vi "Interpolate (single).vi"(8 "error in (no error)":errorcluster, 10 "Configure":T1={"X Low"=0.05, "X High"=0.5, "X Step"=0.01, "Fake Point"=0.05} {"Fake Point" format="%#_6p"; "X Step" format="%#_6p"; "X High" format="%#_6p"; "X Low" format="%#_6p"}, 11 "XY-data":cluster{"X-array":dbl[], "Y-array":dbl[]} {"Y-array" format="%#_6p"}) -> (0 "error out":errorcluster, 3 "Interpolated XY-data out":cluster{"X-array":dbl[], "Y-array":dbl[]} {"Y-array" format="%.2p"; "X-array" format="%.2p"})   [LabVIEW 2019, in "xy_utilities.lvlib"]
doc: "Use this VI to interpolate data and add \"fake\" points outside of the given x array.\n\nThe <b>Configure</b> cluster is used to define:\n<b>X Low</b>: Starting x value for interpolation. May lie outside of the input x array range.\n<b>X High</b>: Ending x value for interpolation. May lie outside of the input x array range.\n<b>X Step</b>: Interpolation value.\n<b>Fake Point</b>: Value added to the y array for x values outside of the x array input range.\n\nWire data to the data input to determine the polymorphic instance to use or manually select the instance."
uses:
  xy_utilities.lvlib
  <vilib>/Analysis/NI_AALBase.lvlib
  <vilib>/Analysis/1siggen.llb/Ramp Pattern by Delta.vi
  <vilib>/gmath/NI_Gmath.lvlib
  Typedefs/Interpolation Configuration--cluster.ctl
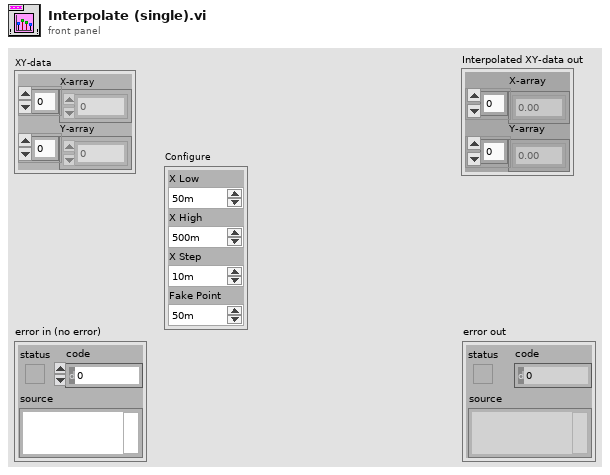
[diagram p1: front panel]
types:
  T1 = typedef "xy_utilities.lvlib/Interpolation Configuration--cluster.ctl" = cluster{"X Low":dbl, "X High":dbl, "X Step":dbl, "Fake Point":dbl}
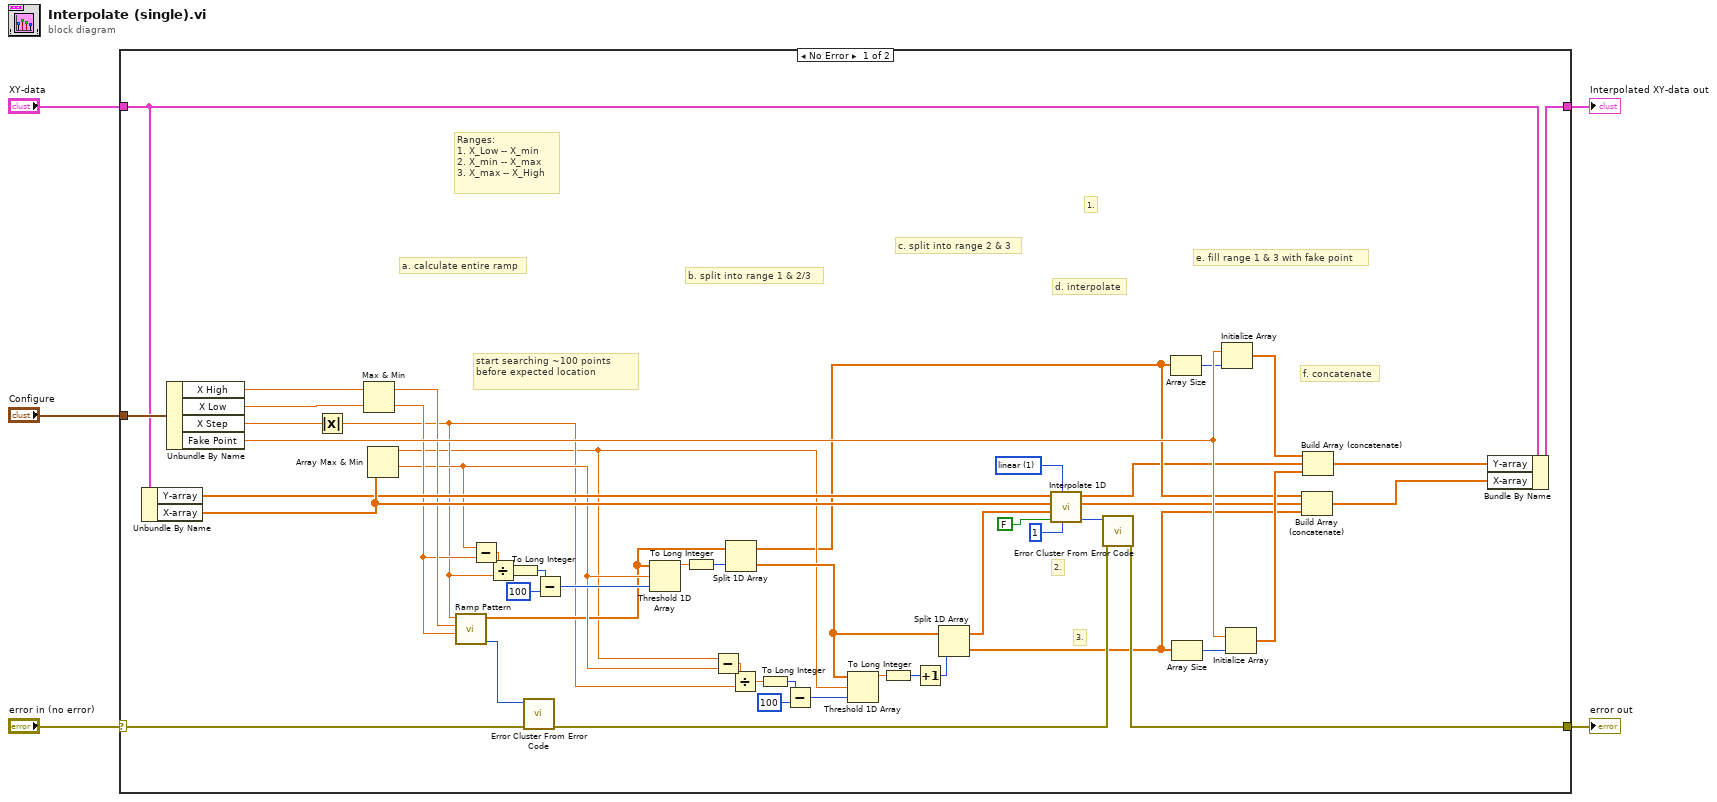
[diagram p0: block diagram]
diagram:
  n1 = case shown="No Error" "error in (no error)" {
    selector: "error in (no error)" -> [w44 w57]
    tunnel: [w43 w57] -> w4
    tunnel: "XY-data" -> [w45 w56]
    tunnel: [w53 w56] -> w1
    tunnel: "Configure" -> [w48 _]
    frame No Error {
      w42 = 1 items=["nearest", "linear", "spline", "cubic Hermite", "Lagrange"] ("method")
      # "f. concatenate"
      # "e. fill range 1 & 3 with fake point"
      # "start searching ~100 points before expected location"
      # "d. interpolate"
      # "c. split into range 2 & 3"
      # "b. split into range 1 & 2/3"
      # "a. calculate entire ramp"
      # "3."
      # "1."
      # "2."
      # "Ranges:\n1. X_Low -- X_min\n2. X_min -- X_max\n3. X_max -- X_High"
      n2 = Unbundle By Name(w45) -> ("Y-array"=w51:dbl[], "X-array"=w55:dbl[])
      n3 = Unbundle By Name(w48) -> ("X High"=w52:dbl, "X Low"=w50:dbl, "X Step"=w49:dbl, "Fake Point"=w54:dbl)
      n4 = Absolute Value(x=w49) -> (abs(x)=w10:dbl)
      n5 = Max & Min(x=w52, y=w50) -> (max(x,y)=w32:dbl, min(x,y)=w28:dbl)
      n6 = Array Max & Min(array=w55) -> (max value=w9:dbl, min value=w16:dbl)  [unwired: 2 out]
      n7 = call-poly <vilib>:"Ramp Pattern.vi"("start"=w28, "end"=w32, "delta"=w10) -> ("error"=w31:i32, "Ramp Pattern"=w11:dbl[])  [unwired: 6 in, 1 out]
      n8 = Subtract(x=w16, y=w28) -> (x-y=w27:dbl)
      n9 = Divide(x=w27, y=w10) -> (x/y=w26:dbl)
      n10 = To Long Integer(number=w26) -> (32bit integer=w14:i32)
      n11 = call <vilib>:"Error Cluster From Error Code.vi"("error in (no error)"=w44, "error code (0)"=w31) -> ("error out"=w38:errorcluster)  [unwired: 7 in]
      n12 = Subtract(x=w14, y=100) -> (x-y=w24:i32)
      n13 = Threshold 1D Array(1:w24, 2:w16, 3:w11) -> (0:w30:dbl)
      n14 = To Long Integer(number=w30) -> (32bit integer=w29:i32)
      n15 = Subtract(x=w9, y=w16) -> (x-y=w17:dbl)
      n16 = Split 1D Array(array=w11, index=w29) -> (first subarray=w8:dbl[], second subarray=w22:dbl[])
      n17 = Divide(x=w17, y=w10) -> (x/y=w18:dbl)
      n18 = To Long Integer(number=w18) -> (32bit integer=w13:i32)
      n19 = Subtract(x=w13, y=100) -> (x-y=w15:i32)
      n20 = Threshold 1D Array(1:w15, 2:w9, 3:w22) -> (0:w23:dbl)
      n21 = To Long Integer(number=w23) -> (32bit integer=w21:i32)
      n22 = Increment(x=w21) -> (x+1=w6:i32)
      n23 = Split 1D Array(array=w22, index=w6) -> (first subarray=w20:dbl[], second subarray=w12:dbl[])
      n24 = call <vilib>:"Interpolate 1D.vi"("ntimes"=1, "method"=w42, "X is monotonic"=FALSE, "xi"=w20, "X"=w55, "Y"=w51) -> ("error"=w40:i32, "xi used"=w33:dbl[], "yi"=w7:dbl[])  [unwired: 3 in]
      n25 = call <vilib>:"Error Cluster From Error Code.vi"("error in (no error)"=w38, "error code (0)"=w40) -> ("error out"=w43:errorcluster)  [unwired: 7 in]
      n26 = Array Size(array=w8) -> (size(s)=w36:i32)
      n27 = Array Size(array=w12) -> (size(s)=w37:i32)
      n28 = Initialize Array(w54, w36) -> (w35:dbl[])
      n29 = Initialize Array(w54, w37) -> (w34:dbl[])
      n30 = Build Array (concatenate)(w8, w33, w12) -> (w46:dbl[])
      n31 = Build Array (concatenate)(w35, w7, w34) -> (w47:dbl[])
      n32 = Bundle By Name(cluster=w45, "Y-array"=w47, "X-array"=w46) -> (w53:cluster{"X-array":dbl[], "Y-array":dbl[]})
    }
    frame Error {
    }
  }
  "error out" <- w4
  "Interpolated XY-data out" <- w1
